vi "Stop Core.vi"(10 "final error code":i32, 11 "Popup ViewManager in":refnum<class "Popup ViewManager.lvclass">) -> (3 "Popup ViewManager out":refnum<class "Popup ViewManager.lvclass">)   [LabVIEW 2017, in "Popup ViewManager.lvlib" / "Popup ViewManager.lvclass"]
doc: "(<B>Filename</B>: Actor Framework.lvlib:Actor.lvclass:Stop Core.vi)\n\nDefines what the actor does before it stops. Use the <B>final error code</B> input to determine whether the actor shut down in response to an error.\n\nBy default, this method does nothing. A descendant class may override it to define behavior, such as shutting down any processes the actor initiated in its override of the Actor Core method.\n\n<License>\nCopyright © 2017 Composed Systems, LLC | All rights reserved\nwww.composed.io\n\nAuthor: Ethan Stern <ethan.stern@composed.io>\n\nThis software is provided \"AS IS\" WITHOUT WARRANTIES, either express or implied, AND IS FOR EDUCATIONAL PURPOSES ONLY.\n</License>"
uses:
  <vilib>/gpm_packages/@cs/popup-viewmanager/Source/Popup ViewManager/Popup ViewManager.lvclass
  <vilib>/gpm_packages/@cs/popup-viewmanager/Source/Popup ViewManager/Popup ViewManager.lvclass/Popup ViewManager.ctl
  <vilib>/ActorFramework/Message Enqueuer/Message Enqueuer.lvclass/Message Enqueuer.ctl
  <vilib>/ActorFramework/Message Enqueuer/Enqueue.vi
  <vilib>/ActorFramework/Stop Msg/Stop Msg.lvclass
  C:/Program Files/National Instruments/LabVIEW 2017/vi.lib/ActorFramework/Message/Message.lvclass
  <vilib>/ActorFramework/Message Priority Queue/Priority Enqueue.vi
  <vilib>/gpm_packages/@cs/mva-dialogbox/source/IDialogBox/IDialogBox/IDialogBox.lvclass
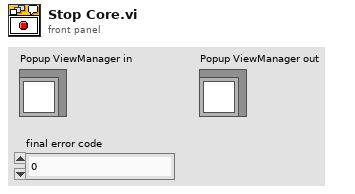
[diagram p1: front panel]
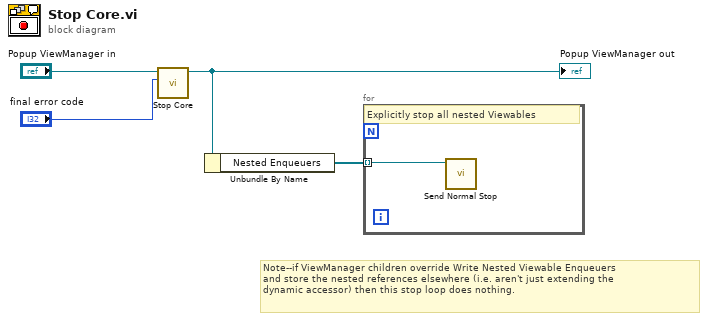
[diagram p0: block diagram]
diagram:
  # "Note--if ViewManager children override Write Nested Viewable Enqueuers\nand store the nested references elsewhere (i.e. aren't just extending the\ndynamic accessor) then this stop loop does nothing."
  n1 = call-parent "Stop Core.vi"("final error code"="final error code", "IDialogBox in"="Popup ViewManager in") -> ("IDialogBox out"=w2:refnum<class "Popup ViewManager.lvclass">)  [unwired: 9 in]
  "Popup ViewManager out" <- w2
  n2 = Unbundle By Name(w2) -> ("Nested Enqueuers"=w1:refnum<class "Message Enqueuer.lvclass">[])
  n3 = for {
    tunnel: w1 -> [w5] mode=indexing
    # "Explicitly stop all nested Viewables"
    n4 = call <vilib>:"Send Normal Stop.vi"("Message Enqueuer"=w5) -> ()  [unwired: 10 in, 1 out]
  }
